vi "add_uint16.vi"   [LabVIEW 2016]
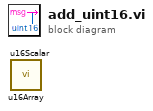
[diagram p0: block diagram]
diagram:
  n1 = call "u16Array.vi"() -> ()  [unwired: 5 in, 1 out]
  n2 = call "u16Scalar.vi"() -> ()  [unwired: 5 in, 1 out]
